vi "MGI Populate Tree with Delimited Strings.vi"(5 "Use Child Only?":bool, 7 "Default Symbol":i32=37, 8 "error in (no error)":errorcluster, 9 "Delimiter":string=".", 10 "Items (Delimited)":string[][](array[string]), 11 "Tree Control":refnum<vi>) -> (0 "error out":errorcluster, 2 "Parents Added":string[](array[string]), 3 "Tree Control Dup":refnum<vi>)   [LabVIEW 2016]
doc: "Populates the specified Tree Control with the specified items. The items are delimited strings where the text of each parent is in the string seperated by delimiters. For example, the string \"C\\Project\\Foo\" with the delimiter \"\\\" would be shown as\nC\n Project\n Foo\nEach Row in the 2D Items array is a child item. The first column contains the Tags. Subsequent columns contain Text for the Tree control columns.\nIf \"Use Child Only Items?\" is true, then items in the 2D array that are not followed by a descendent item are inserted as \"Child Only\". Otherwise, all items are inserted as Child Only=False. NOTE: If Use Child Only Items? is true, then the 2D array must have all parent tags followed immediately by one child item.\n\nAuthored by Shawn D. Walpole\nsupport@mooregoodideas.com\nwww.mooregoodideas.com\n\nCopyright (c) 2010, Moore Good Ideas, Inc.\n\nAll rights reserved.\n\nRedistribution and use in source and binary forms, with or without modification, are permitted provided that the following conditions are met:\n\n * Redistributions of source code must retain the above copyright notice, this list of conditions and the following disclaimer.\n * Redistributions in binary form must reproduce the above copyright notice, this list of conditions and the following disclaimer in the documentation and/or other materials provided with the distribution.\n * Neither the name of Moore Good Ideas, Inc. nor the names of its contributors may be used to endorse or promote products derived from this software without specific prior written permission.\n\nTHIS SOFTWARE IS PROVIDED BY THE COPYRIGHT HOLDERS AND CONTRIBUTORS \"AS IS\" AND ANY EXPRESS OR IMPLIED WARRANTIES, INCLUDING, BUT NOT LIMITED TO, THE IMPLIED WARRANTIES OF MERCHANTABILITY AND FITNESS FOR A PARTICULAR PURPOSE ARE DISCLAIMED. IN NO EVENT SHALL THE COPYRIGHT OWNER OR CONTRIBUTORS BE LIABLE FOR ANY DIRECT, INDIRECT, INCIDENTAL, SPECIAL, EXEMPLARY, OR CONSEQUENTIAL DAMAGES (INCLUDING, BUT NOT LIMITED TO, PROCUREMENT OF SUBSTITUTE GOODS OR SERVICES; LOSS OF USE, DATA, OR PROFITS; OR BUSINESS INTERRUPTION) HOWEVER CAUSED AND ON ANY THEORY OF LIABILITY, WHETHER IN CONTRACT, STRICT LIABILITY, OR TORT (INCLUDING NEGLIGENCE OR OTHERWISE) ARISING IN ANY WAY OUT OF THE USE OF THIS SOFTWARE, EVEN IF ADVISED OF THE POSSIBILITY OF SUCH DAMAGE."
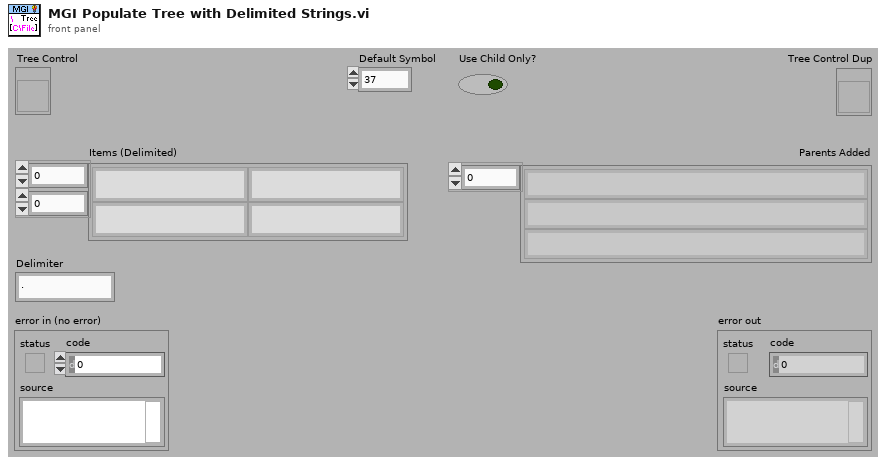
[diagram p1: front panel]
types:
  T1 = cluster{"Left Cell String":string, "Child Text":string[], "Child Tag":string, "Item Indent":i32, "Child Only?":bool, "Glyph Index":i32}[]
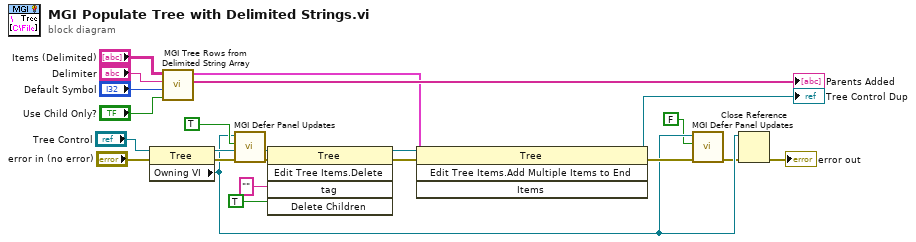
[diagram p0: block diagram]
diagram:
  n1 = property class="Tree"(reference="Tree Control", error in="error in (no error)") -> (reference out=w8:refnum<vi>, error out=w7:errorcluster, "Owning VI"=w4:refnum<vi>)
  n2 = call <userlib>:"MGI Tree Rows from Delimited String Array.vi"("Use Child Only? (False)"="Use Child Only?", "Default Symbol"="Default Symbol", "Delimiter"="Delimiter", "Items (Delimited)"="Items (Delimited)") -> ("Parent Tag Added[]"=→"Parents Added":string[], "Item to Add[]"=w11:T1)  [unwired: 6 in]
  n3 = call <userlib>:"MGI Defer Panel Updates.vi"("Error In"=w7, "Defer Updates?"=TRUE ("Defer Panel Updates"), "VI Reference (Caller)"=w4) -> ("Error Out"=w10:errorcluster)  [unwired: 8 in]
  n4 = invoke on="Invoke Node" class="Tree" method="Edit Tree Items.Delete"(reference=w8, error in=w10, "tag"="" ("Tag"), "Delete Children"=TRUE ("Delete Children?")) -> (reference out=w13:refnum<vi>, error out=w12:errorcluster)  [unwired: 1 in, 3 out]
  n5 = invoke on="Invoke Node" class="Tree" method="Edit Tree Items.Add Multiple Items to End"(reference=w13, error in=w12, "Items"=w11) -> (reference out=→"Tree Control Dup":refnum<vi>, error out=w6:errorcluster)  [unwired: 1 in, 2 out]
  n6 = call <userlib>:"MGI Defer Panel Updates.vi"("Error In"=w6, "Defer Updates?"=FALSE ("Defer Panel Updates"), "VI Reference (Caller)"=w4) -> ("Error Out"=w1:errorcluster)  [unwired: 8 in]
  n7 = Close Reference(reference=w4, error in (no error)=w1) -> (error out=→"error out":errorcluster)
